vi "CloseBuild.vi"(8 "error in (no error)":errorcluster, 9 "GeneratedFiles":path[](array[path]), 10 "GeneratedDirectories":path[](array[path]), 11 "Class in":refnum<class "Installer.lvclass">) -> (0 "error out":errorcluster, 1 "GeneratedFiles out":path[](array[path]), 3 "Class out":refnum<class "Installer.lvclass">)   [LabVIEW 2020, in "Installer.lvclass"]
uses:
  <vilib>/AppBuilder/IB_Classes/Installer/Installer.lvclass
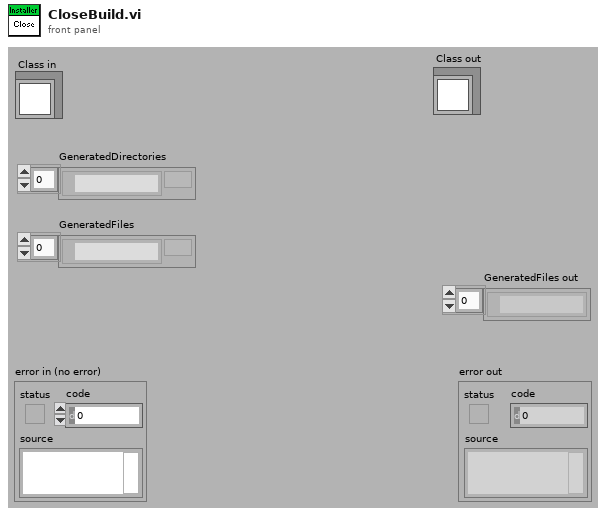
[diagram p1: front panel]
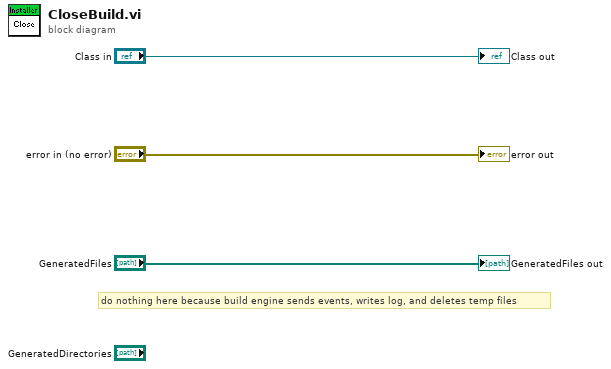
[diagram p0: block diagram]
diagram:
  # "do nothing here because build engine sends events, writes log, and deletes temp files"
  "error out" <- "error in (no error)"
  "GeneratedFiles out" <- "GeneratedFiles"
  "Class out" <- "Class in"
